vi "Execute.vi"(8 "error in (no error)":errorcluster, 11 "Decorator in":refnum<class "Decorator.lvclass">) -> (0 "error out":errorcluster, 2 "Data":dbl[](array[numeric]), 3 "Decorator out":refnum<class "Decorator.lvclass">)   [LabVIEW 2021, in "Decorator.lvclass"]
uses:
  Decorator.lvclass
  Decorator.lvclass/Decorator.ctl
  Component/Component.lvclass
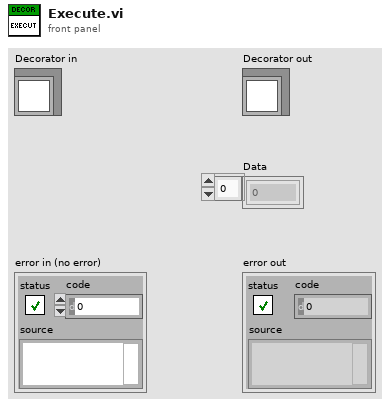
[diagram p1: front panel]
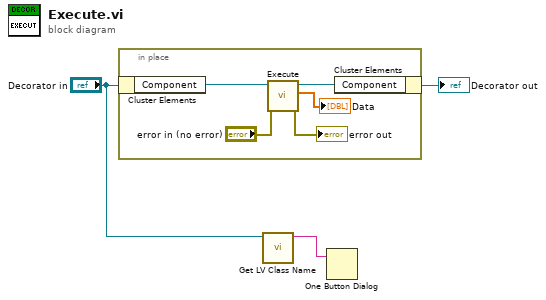
[diagram p0: block diagram]
diagram:
  n1 = in-place {
    n2 = in-place-cluster #1("Decorator in") -> ("Component"=w5:refnum<class "Component.lvclass">)
    n3 = call-dynamic "Execute.vi"("error in (no error)"="error in (no error)", "Data Source in"=w5) -> ("error out"=→"error out":errorcluster, "Data"=→"Data":dbl[], "Data Source out"=w4:refnum<class "Component.lvclass">)  [unwired: 7 in]
    n4 = in-place-cluster #1("Component"=w4) -> (→"Decorator out":refnum<class "Decorator.lvclass">)
  }
  n5 = call <vilib>:"Get LV Class Name.vi"("object"="Decorator in") -> ("class name"=w1:string)  [unwired: 9 in, 1 out]
  n6 = One Button Dialog(message=w1) -> ()  [unwired: 1 in, 1 out]
